vi "Pytheorem.vi"(9 "C":dbl, 10 "B":dbl, 11 "A":dbl) -> (1 "C Output":dbl, 2 "B Output":dbl, 3 "A Output":dbl)   [LabVIEW 2017]
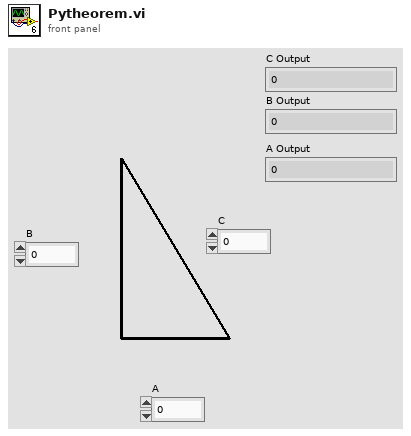
[diagram p1: front panel]
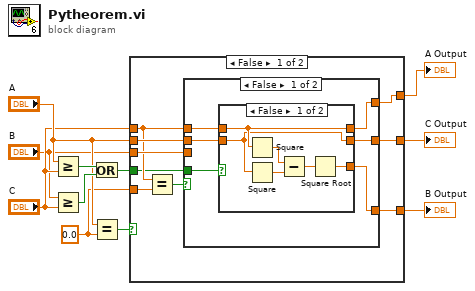
[diagram p0: block diagram]
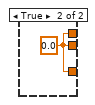
[diagram p2: hidden frame]
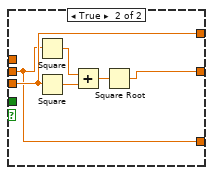
[diagram p3: hidden frame]
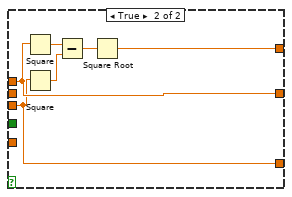
[diagram p4: hidden frame]
diagram:
  w1 = 0.0 ("y")
  n1 = Greater Or Equal?(x="A", y="C") -> (x >= y?=w10:bool)
  n2 = Greater Or Equal?(x="B", y="C") -> (x >= y?=w9:bool)
  n3 = Or(x=w10, y=w9) -> (x .or. y?=w8:bool)
  n4 = Equal?(x="A", y=w1) -> (x = y?=w11:bool)
  n5 = case shown="False" w11 {
    tunnel: "B" -> [w17 w40]
    tunnel: "C" -> [w13 w41]
    tunnel: [w15 w42] -> w7
    tunnel: [w16 w41] -> w6
    tunnel: [w14 w40] -> w5
    tunnel: w1 -> [w20 _]
    tunnel: "A" -> [w18 _]
    tunnel: w8 -> [w12 _]
    frame False {
      n6 = Equal?(x=w13, y=w20) -> (x = y?=w19:bool)
      n7 = case shown="False" w19 {
        tunnel: w18 -> [w25 w34]
        tunnel: w17 -> [_ w35]
        tunnel: [w21 w36] -> w16
        tunnel: [w22 w35] -> w15
        tunnel: [w26 w34] -> w14
        tunnel: w13 -> [w24 _]
        tunnel: w12 -> [w23 _]
        frame False {
          n8 = case shown="False" w23 {
            tunnel: [w29 w33] -> w26
            tunnel: w25 -> [w27 _]
            tunnel: w24 -> [w28 _]
            tunnel: [w28 w33] -> w22
            tunnel: [w27 w33] -> w21
            frame False {
              n9 = Square(x=w28) -> (x^2=w32:dbl)
              n10 = Square(x=w27) -> (x^2=w31:dbl)
              n11 = Subtract(x=w32, y=w31) -> (x-y=w30:dbl)
              n12 = Square Root(x=w30) -> (sqrt(x)=w29:dbl)
            }
            frame True {
              w33 = 0.0
            }
          }
        }
        frame True {
          n13 = Square(x=w34) -> (x^2=w39:dbl)
          n14 = Square(x=w35) -> (x^2=w38:dbl)
          n15 = Add(x=w39, y=w38) -> (x+y=w37:dbl)
          n16 = Square Root(x=w37) -> (sqrt(x)=w36:dbl)
        }
      }
    }
    frame True {
      n17 = Square(x=w41) -> (x^2=w45:dbl)
      n18 = Square(x=w40) -> (x^2=w44:dbl)
      n19 = Subtract(x=w45, y=w44) -> (x-y=w43:dbl)
      n20 = Square Root(x=w43) -> (sqrt(x)=w42:dbl)
    }
  }
  "A Output" <- w7
  "B Output" <- w5
  "C Output" <- w6
